vi "Keithley6485 Bkg Check.vi"(8 "error in":errorcluster, 11 "VISA in":refnum<visa-resource-name>="COM3") -> (0 "error out":errorcluster, 2 "Zero Offset":string, 3 "VISA out":refnum<visa-resource-name>)   [LabVIEW 2018]
panel:
  in  "Zero Check Procedure":string=":TRIG:COUN 1;:SYST:ZCH 1;:CURR:RANG 2E-9;:INIT;:SYST:ZCOR 0;:SYST:ZCOR:ACQ;:SYST:ZCH 0;:SYST:ZCOR 1;:CURR:RANG:AUTO 1;:FETC?"
  # "Error out reports Serial I/O errors.\n\nKeithley Error reports error messages returned by the Keithley 6485 picoAmmeter.  Currently, only overvoltage and invalid data errors are supported by this VI."
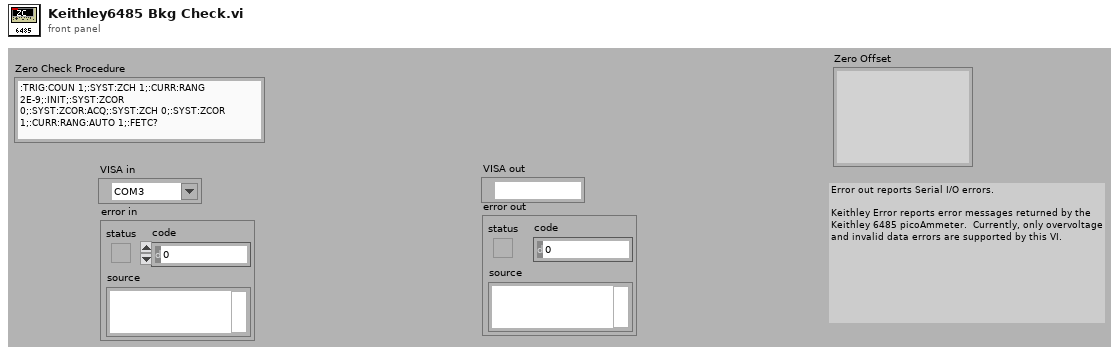
[diagram p1: front panel]
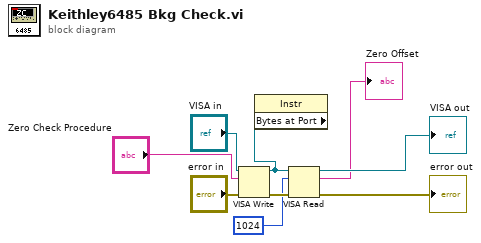
[diagram p0: block diagram]
diagram:
  n1 = VISA Write(VISA resource name="VISA in", write buffer="Zero Check Procedure", error in (no error)="error in") -> (VISA resource name out=w5:refnum<visa-resource-name>, error out=w6:errorcluster)  [unwired: 1 out]
  n2 = property class="Instr" props=["Bytes at Port"](reference=w5) -> ()  [unwired: 1 in, 3 out]
  n3 = VISA Read(VISA resource name=w5, byte count=u32 1024, error in (no error)=w6) -> (VISA resource name out=→"VISA out":refnum<visa-resource-name>, read buffer=→"Zero Offset":string, error out=→"error out":errorcluster)  [unwired: 1 out]
